vi "Parse Waveform.vi"(10 "Waveform":waveform(dbl)) -> (0 "Y":dbl[](array[numeric]), 1 "dt":dbl, 2 "t0":timestamp, 4 "attributes":variant)   [LabVIEW 2021]
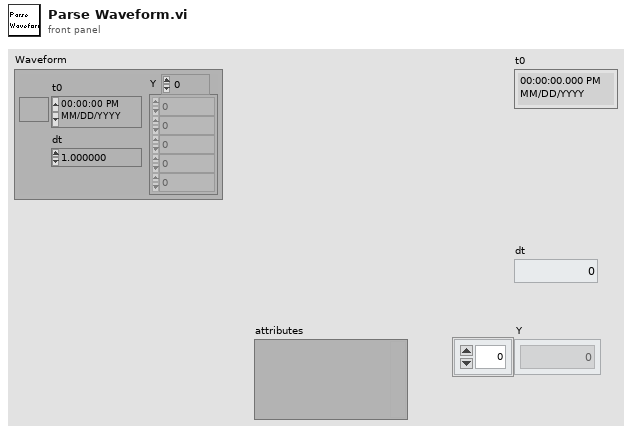
[diagram p1: front panel]
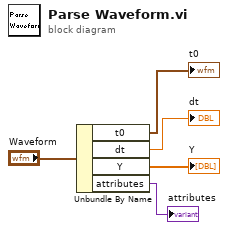
[diagram p0: block diagram]
diagram:
  n1 = Unbundle By Name("Waveform") -> ("t0"=→"t0":timestamp, "dt"=→"dt":dbl, "Y"=→"Y":dbl[], "attributes"=→"attributes":variant)
